vi "initializeCameraAndSetResolution.vi"(8 "error in":errorcluster, 11 "seesion in":T1) -> (0 "error out":errorcluster, 1 "mode names":string[](array[string]), 2 "modes":u32[](array[numeric]), 3 "session out":T1 caption="Session Out", 4 "current mode":u32)   [LabVIEW 2024]
uses:
  <vilib>/userDefined/High Color/IMAQdx.ctl
  <vilib>/vision/driver/NI_Vision_Acquisition_Software.lvlib
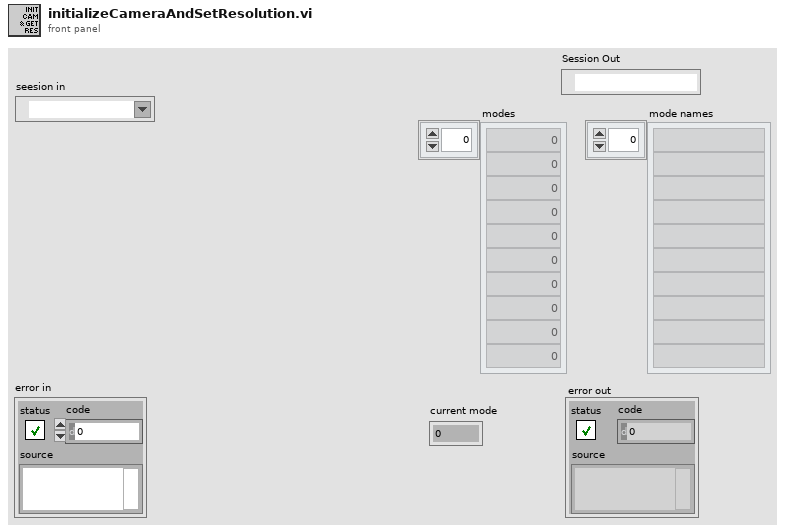
[diagram p1: front panel]
types:
  T1 = typedef "IMAQdx.ctl" = refnum<k21>
  T2 = cluster{"Video Mode":u32, "Video Mode Name":string}[]
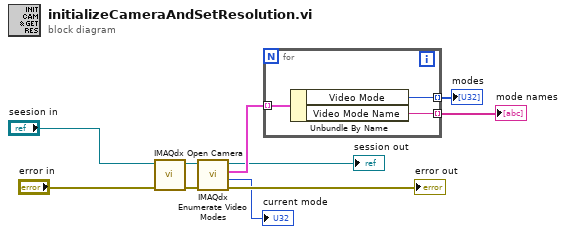
[diagram p0: block diagram]
diagram:
  n1 = call <vilib>:"IMAQdx Open Camera.vi"("error in"="error in", "Session In"="seesion in") -> ("error out"=w10:errorcluster, "Session Out"=w9:T1)  [unwired: 8 in]
  n2 = call <vilib>:"IMAQdx Enumerate Video Modes.vi"("error in"=w10, "Session In"=w9) -> ("error out"=→"error out":errorcluster, "Current Mode"=→"current mode":u32, "Video Modes"=w6:T2, "Session Out"=→"session out":T1)  [unwired: 6 in]
  n3 = for {
    tunnel: w6 -> [w13] mode=indexing
    tunnel: [w12] -> w5 mode=indexing
    tunnel: [w11] -> w4 mode=indexing
    n4 = Unbundle By Name(w13) -> ("Video Mode"=w12:u32, "Video Mode Name"=w11:string)
  }
  "modes" <- w5
  "mode names" <- w4
